vi "client send data for server.vi"() -> ()   [LabVIEW 2020]
panel:
  in  "Data in":string[](array[string])
  out "?":errorcluster
  in  "?":errorcluster
  in  "IP address":string
  out "Respone Led":bool
  in  "Send Data Button":bool
  in  "Stop Send Data":bool
  in  "Port 1":u16
  in  "Port 2":u16
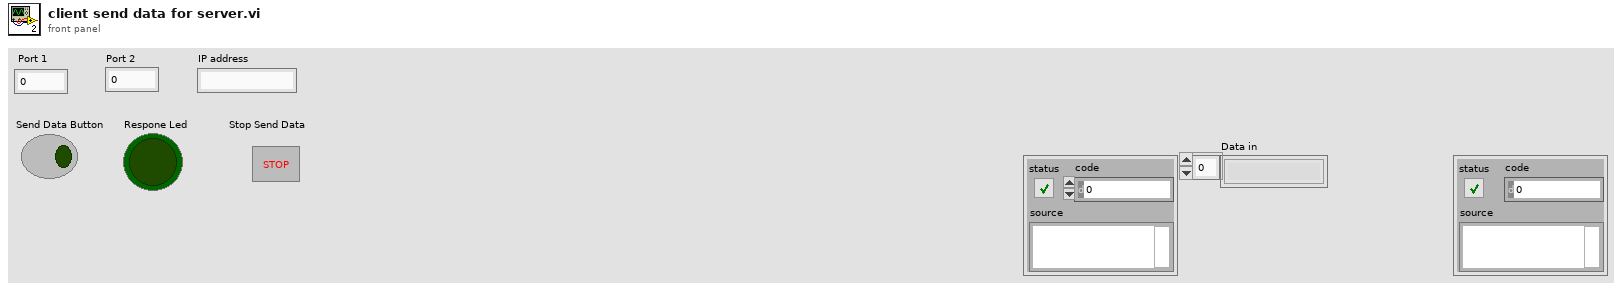
[diagram p1: front panel]
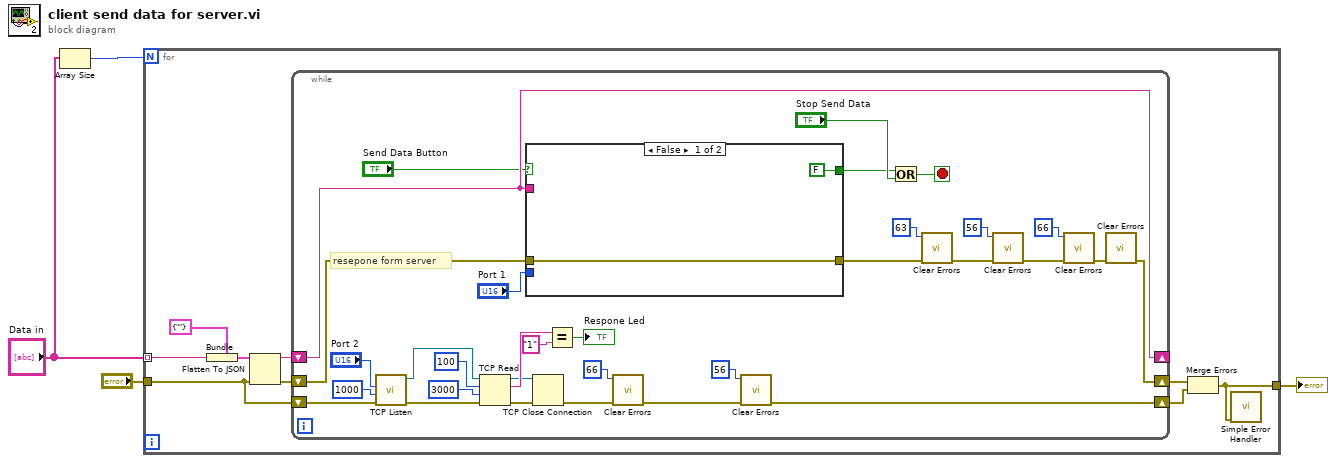
[diagram p0: block diagram]
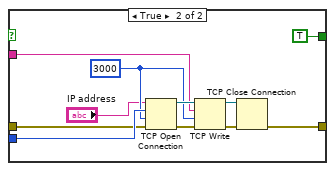
[diagram p2: hidden frame]
diagram:
  n1 = Array Size(array="Data in") -> (size(s)=w4:i32)
  n2 = for {
    N: w4 -> [_]
    tunnel: "Data in" -> [w10] mode=indexing
    tunnel: [w6] -> w2
    tunnel: "?" -> [w5]
    n3 = Bundle(cluster=cluster{"Message":string} {"Message"=""}, "Message"=w10) -> (w11:cluster{"Message":string})
    n4 = Flatten To JSON(anything=w11, error in (no error)=w5) -> (JSON string=w9:string, 11:w8:errorcluster)  [unwired: 1 in]
    n5 = while {
      shift-right: [w34] -> _
      shift-left: w9 -> [w34]
      shift-right: [w41] -> w7
      shift-left: w5 -> [w42]
      shift-right: [w18] -> w13
      shift-left: w8 -> [w40]
      stop <- w15 stop-if-true
      # "resepone form server"
      n6 = call <vilib>:"TCP Listen.vi"("error in (no error)"=w42, "timeout ms (wait forever: -1)"=1000, "port"="Port 2") -> ("error out"=w30:errorcluster, "connection ID"=w29:refnum<k5>)  [unwired: 4 in, 3 out]
      n7 = TCP Read(connection ID=w29, bytes to read=100, error in (no error)=w30, 9:3000 ("timeout ms (25000)")) -> (connection ID out=w27:refnum<k5>, data out=w44:string, error out=w28:errorcluster)  [unwired: 1 in]
      n8 = case shown="False" "Send Data Button" {
        tunnel: w34 -> [_ w54]
        tunnel: [w47 w50] -> w33
        tunnel: "Port 1" -> [_ w53]
        tunnel: w40 -> [w47 w52]
        tunnel: [FALSE TRUE] -> w23
        frame False {
        }
        frame True {
          w51 = 3000 ("timeout ms (60000)")
          n9 = TCP Open Connection(address="IP address", remote port or service name=w53, timeout ms (60000)=w51, error in (no error)=w52) -> (connection ID=w55:refnum<k5>, error out=w58:errorcluster)  [unwired: 1 in]
          n10 = TCP Write(connection ID=w55, data in=w54, error in (no error)=w58, 9:w51) -> (connection ID out=w56:refnum<k5>, error out=w57:errorcluster)  [unwired: 1 out]
          n11 = TCP Close Connection(connection ID=w56, error in (no error)=w57) -> (error out=w50:errorcluster)  [unwired: 1 in, 1 out]
        }
      }
      n12 = TCP Close Connection(connection ID=w27, error in (no error)=w28) -> (error out=w38:errorcluster)  [unwired: 1 in, 1 out]
      n13 = Equal?(x=w44, y="1") -> (x = y?=→"Respone Led":bool)
      n14 = call <vilib>:"Clear Errors.vi"("error in (no error)"=w38, "specific error code to clear (0: all)"=66) -> ("error out"=w37:errorcluster)  [unwired: 4 in, 1 out]
      n15 = call <vilib>:"Clear Errors.vi"("error in (no error)"=w37, "specific error code to clear (0: all)"=56) -> ("error out"=w41:errorcluster)  [unwired: 4 in, 1 out]
      n16 = Or(x=w23, y="Stop Send Data") -> (x .or. y?=w15:bool)
      n17 = call <vilib>:"Clear Errors.vi"("error in (no error)"=w33, "specific error code to clear (0: all)"=63) -> ("error out"=w22:errorcluster)  [unwired: 4 in, 1 out]
      n18 = call <vilib>:"Clear Errors.vi"("error in (no error)"=w22, "specific error code to clear (0: all)"=56) -> ("error out"=w21:errorcluster)  [unwired: 4 in, 1 out]
      n19 = call <vilib>:"Clear Errors.vi"("error in (no error)"=w21, "specific error code to clear (0: all)"=66) -> ("error out"=w19:errorcluster)  [unwired: 4 in, 1 out]
      n20 = call <vilib>:"Clear Errors.vi"("error in (no error)"=w19) -> ("error out"=w18:errorcluster)  [unwired: 5 in, 1 out]
    }
    n21 = Merge Errors(w13, w7) -> (w6:errorcluster)
    n22 = call <vilib>:"Simple Error Handler.vi"("error in (no error)"=w6) -> ()  [unwired: 4 in, 5 out]
  }
  "?" <- w2
